vi "Coerce Sample Size Down.vi"(3 "Bytes Per Sample (B)":u64, 6 "Coerce To (B)":u64, 7 "Size (samples)":u64) -> (1 "Coerced Size (samples)":u64)   [LabVIEW 2016]
doc: "This SubVI coerces a number of samples to be a multiple of the hard disk sector size divided the number of bytes per sample. The Coerced Size will be less than or equal to the Requested size."
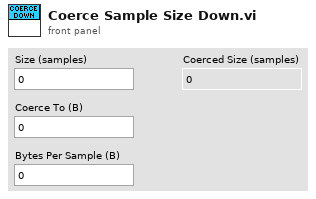
[diagram p1: front panel]
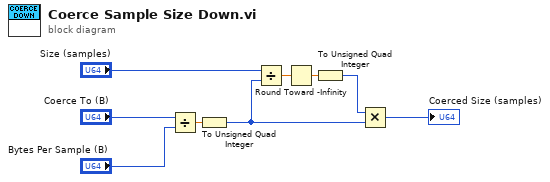
[diagram p0: block diagram]
diagram:
  n1 = Divide(x="Coerce To (B)", y="Bytes Per Sample (B)") -> (x/y=w6:dbl)
  n2 = To Unsigned Quad Integer(1:w6) -> (0:w7:u64)
  n3 = Divide(x="Size (samples)", y=w7) -> (x/y=w3:dbl)
  n4 = Round Toward -Infinity(1:w3) -> (0:w2:dbl)
  n5 = To Unsigned Quad Integer(1:w2) -> (0:w1:u64)
  n6 = Multiply(x=w1, y=w7) -> (x*y=→"Coerced Size (samples)":u64)
